vi "Common Select Readings.vi"(9 "Selected Readings":u32[](array[numeric]), 11 "Readings":dbl[](array[numeric])) -> (3 "Readings Subset":dbl[](array[numeric]))   [LabVIEW 2011, in "Common VIs.lvlib"]
doc: "Selects from the complete beam position vector the BPM readings which are being used to FOFB."
uses:
  Common VIs.lvlib
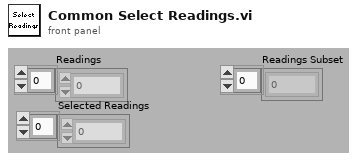
[diagram p1: front panel]
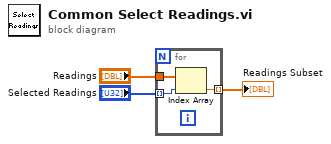
[diagram p0: block diagram]
diagram:
  n1 = for {
    tunnel: "Selected Readings" -> [w5] mode=indexing
    tunnel: "Readings" -> [w6]
    tunnel: [w4] -> w1 mode=indexing
    n2 = Index Array(array=w6, index=w5) -> (element=w4:dbl)
  }
  "Readings Subset" <- w1
